vi "WPI_MotorControlOpen&ConfigurePWM.vi"(5 "PWMPeriodMultiplier":T1 items=["1X"=0, "2X"=1, "4X"=3], 7 "Invert":bool, 8 "error in (no error)":errorcluster, 9 "DeadBand (ms)":T2, 10 "PWM Channel":T5) -> (0 "error out":errorcluster, 3 "MotorControlDeviceRef":T3={"DeviceStatus"={"status"=FALSE, "code"=0, "source"=""}, "Type"=enum."PWM", "PWM"={"PWM Channel"=enum."Invalid", "DeadBand"={"Name"="", "maxPositivePwm"=0, "minPositivePwm"=0, "centerPwm"=0, "maxNegativePwm"=0, "minNegativePwm"=0, "angularRange"=0}}, "CAN"={"Device Number"=0, "SetOutput VI Ref"=variant(refnum<vi> refnum), "GetOutput VI Ref"=variant(refnum<vi> refnum), "Enable VI Ref"=variant(refnum<vi> refnum), "Disable VI Ref"=variant(refnum<vi> refnum), "Data"=variant}, "Invert"=FALSE, "DIO PWM"={"PWM \"Enable\" Channel"=enum."Invalid", "DIOChannel"=enum."Invalid", "PWM Rate"=0.0}})   [LabVIEW 2025]
doc: "This software is licensed. Open the labview\\readme\\WPI Robotics Library Open Source License.txt file for more information."
uses:
  <vilib>/Rock Robotics/SystemInterfaces/DIO/FPGA_DIOPWMChannel.ctl
  <vilib>/Rock Robotics/WPI/MotorControl/WPI_MotorControlDeviceRef.ctl
  <vilib>/Rock Robotics/WPI/MotorControl/WPI_MotorControlType.ctl
  <vilib>/Rock Robotics/WPI/PWM/WPI_PWMDeadband.ctl
  <vilib>/Rock Robotics/SystemInterfaces/DIO/FPGA_DIOChannel.ctl
  <vilib>/Rock Robotics/WPI/PWM/WPI_PWMDeadband_ms.ctl
  <vilib>/Rock Robotics/WPI/PWM/WPI_PWMPeriodMultiplier.ctl
  <vilib>/Rock Robotics/WPI/PWM/WPI_PWMChannelCacheOp.ctl
  <instrlib>/DC Motor Controller/HAIOL/Simulator/DC Motor Controller Simulator.lvclass
  <vilib>/robotics/Simulator/Engine/ctl/DeviceID.ctl
  <vilib>/robotics/Simulator/NI_Robotics_Simulator.lvlib
panel:
  # "On default the deadband\nset is for the full range \nof the PWM motor \nwith 128 at the center."
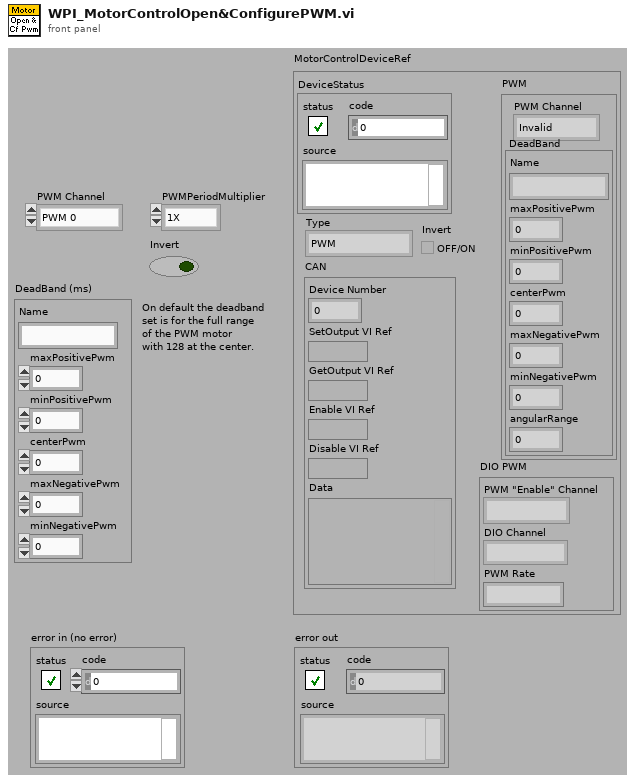
[diagram p1: front panel]
types:
  T1 = typedef "WPI_PWMPeriodMultiplier.ctl" = u8
  T2 = typedef "WPI_PWMDeadband_ms.ctl" = cluster{"Name":string, "maxPositivePwm":dbl, "minPositivePwm":dbl, "centerPwm":dbl, "maxNegativePwm":dbl, "minNegativePwm":dbl}
  T3 = typedef "WPI_MotorControlDeviceRef.ctl" = cluster{"DeviceStatus":errorcluster, "Type":T4, "PWM":cluster{"PWM Channel":T5, "DeadBand":T6}, "CAN":cluster{"Device Number":u8, "SetOutput VI Ref":variant, "GetOutput VI Ref":variant, "Enable VI Ref":variant, "Disable VI Ref":variant, "Data":variant}, "Invert":bool, "DIO PWM":cluster{"PWM \"Enable\" Channel":T5, "DIOChannel":T7, "PWM Rate":dbl}}
  T4 = typedef "WPI_MotorControlType.ctl" = enum16{"PWM", "CAN", "DIO PWM"}
  T5 = typedef "FPGA_DIOPWMChannel.ctl" = enum8{"PWM 0", "PWM 1", "PWM 2", "PWM 3", "PWM 4", "PWM 5", "PWM 6", "PWM 7", "PWM 8", "PWM 9", "PWM MXP 0", "PWM MXP 1", "PWM MXP 2", "PWM MXP 3", "PWM MXP 4", "PWM MXP 5", "PWM MXP 6", "PWM MXP 7", "PWM MXP 8", "PWM MXP 9", "Invalid"}
  T6 = typedef "WPI_PWMDeadband.ctl" = cluster{"Name":string, "maxPositivePwm":i32, "minPositivePwm":i32, "centerPwm":i32, "maxNegativePwm":i32, "minNegativePwm":i32, "angularRange":u16}
  T7 = typedef "FPGA_DIOChannel.ctl" = enum8{"DIO 0", "DIO 1", "DIO 2", "DIO 3", "DIO 4", "DIO 5", "DIO 6", "DIO 7", "DIO 8", "DIO 9", "DIO MXP 0", "DIO MXP 1", "DIO MXP 2", "DIO MXP 3", "DIO MXP 4", "DIO MXP 5", "DIO MXP 6", "DIO MXP 7", "DIO MXP 8", "DIO MXP 9", "DIO MXP 10", "DIO MXP 11", "DIO MXP 12", "DIO MXP 13", "DIO MXP 14", "DIO MXP 15", "SPI Port CS1", "SPI Port CS2", "SPI Port CS3", "SPI Port MISO", "SPI Port MOSI", "Invalid"}
  T8 = typedef "WPI_PWMChannelCacheOp.ctl" = enum16{"Acquire", "Release", "Status"}
  T9 = typedef "NI_Robotics_Simulator.lvlib/DeviceID.ctl" = cluster{"robot ID":string, "sensor/actuator ID":string}
  T10 = typedef "WPI_PWMDeviceRef.ctl" = cluster{"DeviceStatus":errorcluster, "PWM Channel":T5}
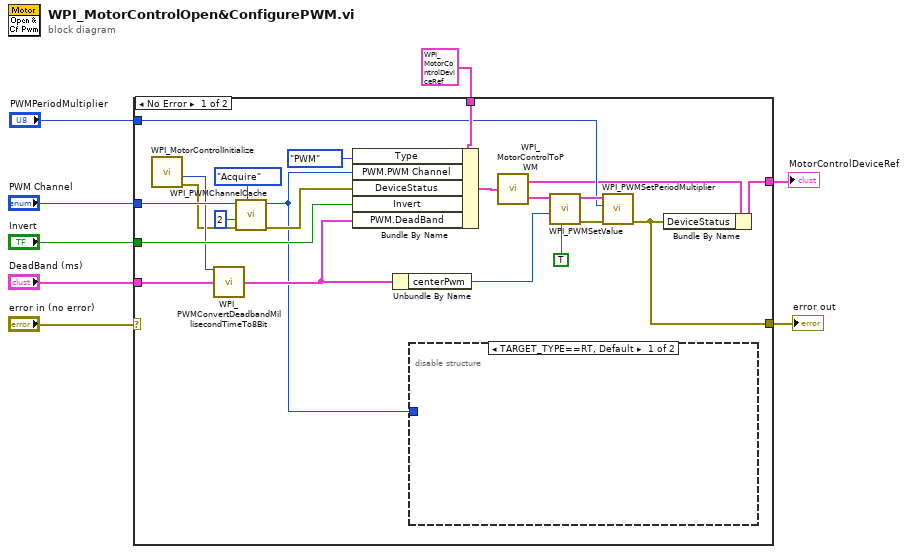
[diagram p0: block diagram]
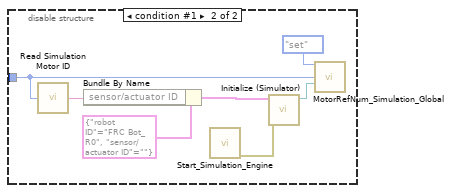
[diagram p2: hidden frame]
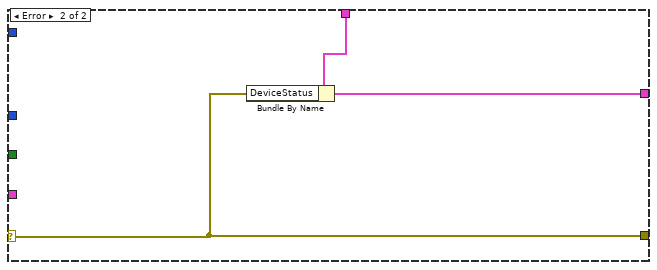
[diagram p3: hidden frame]
diagram:
  n1 = case shown="No Error" "error in (no error)" {
    selector: "error in (no error)" -> [_ w38]
    tunnel: "PWM Channel" -> [w27 _]
    tunnel: T3 {"DeviceStatus"={"status"=FALSE, "code"=0, "source"=""}, "Type"=enum."PWM", "PWM"={"PWM Channel"=enum."PWM 0", "DeadBand"={"Name"="", "maxPositivePwm"=0, "minPositivePwm"=0, "centerPwm"=0, "maxNegativePwm"=0, "minNegativePwm"=0, "angularRange"=0}}, "CAN"={"Device Number"=0, "SetOutput VI Ref"=variant(refnum<vi> refnum), "GetOutput VI Ref"=variant(refnum<vi> refnum), "Enable VI Ref"=variant(refnum<vi> refnum), "Disable VI Ref"=variant(refnum<vi> refnum), "Data"=variant}, "Invert"=FALSE, "DIO PWM"={"PWM \"Enable\" Channel"=enum."Invalid", "DIOChannel"=enum."Invalid", "PWM Rate"=0.0}} ("MotorControlDeviceRef") -> [w29 w40]
    tunnel: [w23 w39] -> w5
    tunnel: [w20 w38] -> w4
    tunnel: "DeadBand (ms)" -> [w17 _]
    tunnel: "Invert" -> [w25 _]
    tunnel: "PWMPeriodMultiplier" -> [w19 _]
    frame No Error {
      n2 = call <vilib>:"WPI_MotorControlInitialize.vi"() -> ("error out"=w10:errorcluster, "LoopTiming"=w11:u16)  [unwired: 10 in]
      n3 = call <vilib>:"WPI_PWMConvertDeadbandMillisecondTimeTo8Bit.vi"("DIO Loop Timing (ticks)"=w11, "PWMDeadband (ms)"=w17) -> ("PWMDeadband Coefficient"=w16:T6)  [unwired: 13 in]
      n4 = call <vilib>:"WPI_PWMChannelCache.vi"("Operation"=WPI_PWMChannelCacheOp."Acquire", "error in (no error)"=w10, "Additional Depth"=2, "PWMChannel"=w27) -> ("error out"=w28:errorcluster, "AllocatedPWMChannel"=w9:T5)  [unwired: 1 in, 5 out]
      n5 = Bundle By Name(cluster=w29, "Type"=WPI_MotorControlType."PWM", "PWM.PWM Channel"=w9, "DeviceStatus"=w28, "Invert"=w25, "PWM.DeadBand"=w16) -> (w15:T3)
      n6 = Unbundle By Name(w16) -> ("centerPwm"=w26:i32)
      n7 = disable-structure shown="TARGET_TYPE==RT, Default" {
        disable-tunnel: w9 -> [_ w31]
        frame condition #0 (active) {
        }
        frame condition #1 {
          n8 = call <vilib>:"Read Simulation Motor ID.vi"("PWM.PWM Channel"=w31) -> ("motor ID"=w36:string)  [unwired: 13 in, 1 out]
          n9 = Bundle By Name(cluster=T9 {"robot ID"="FRC Bot_R0", "sensor/actuator ID"=""} ("Device ID"), "sensor/actuator ID"=w36) -> (w35:T9)
          n10 = call <vilib>:"Start_Simulation_Engine.vi"() -> ("error out"=w34:errorcluster)  [unwired: 15 in]
          n11 = call <instrlib>:"Initialize (Simulator).vi"("error in (no error)"=w34, "Device ID"=w35) -> ("DC Motor Controller out"=w33:refnum<class "DC Motor Controller.lvclass">)  [unwired: 8 in, 1 out]
          n12 = call <vilib>:"MotorRefNum_Simulation_Global.vi"("menu"=enum16{"set", "get", "delete"}."set", "PWM Channel"=w31, "DC Motor Controller Set"=w33) -> ()  [unwired: 11 in, 2 out]
        }
      }
      n13 = call <vilib>:"WPI_MotorControlToPWM.vi"("MotorControlDeviceRef"=w15) -> ("MotorControlDeviceRef"=w14:T3, "PWMDeviceRef"=w24:T10)
      n14 = call <vilib>:"WPI_PWMSetValue.vi"("Indicate Zero"=TRUE, "Value"=w26, "PWMDeviceRef"=w24) -> ("error out"=w21:errorcluster, "PWMDeviceRef"=w22:T10)  [unwired: 1 in, 6 out]
      n15 = call <vilib>:"WPI_PWMSetPeriodMultiplier.vi"("error in (no error)"=w21, "PWMPeriodMultiplier"=w19, "PWMDeviceRef"=w22) -> ("error out"=w20:errorcluster)  [unwired: 8 out]
      n16 = Bundle By Name(cluster=w14, "DeviceStatus"=w20) -> (w23:T3)
    }
    frame Error {
      n17 = Bundle By Name(cluster=w40, "DeviceStatus"=w38) -> (w39:T3)
    }
  }
  "MotorControlDeviceRef" <- w5
  "error out" <- w4
